vi "GetMatchNum.vi"(7 "Update?":bool, 8 "MatchNumberIn":u16) -> (3 "MatchNumberOut":u16)   [LabVIEW 2017]
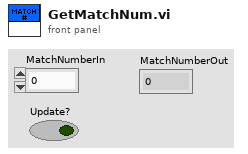
[diagram p1: front panel]
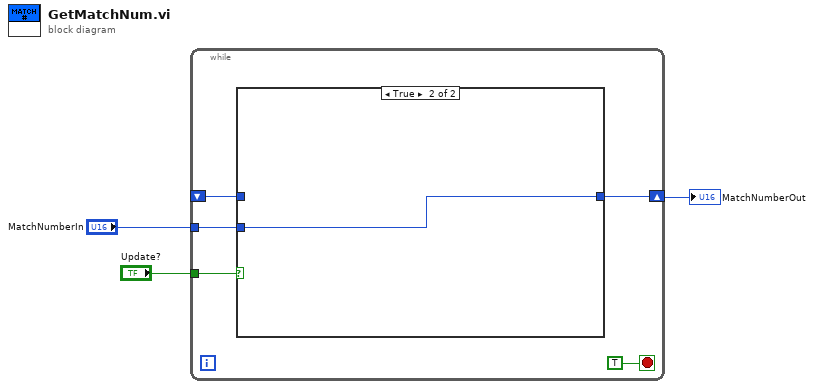
[diagram p0: block diagram]
diagram:
  n1 = while {
    shift-right: [w7] -> w1
    shift-left: _ -> [w8]
    tunnel: "MatchNumberIn" -> [w6]
    tunnel: "Update?" -> [w5]
    stop <- TRUE stop-if-true
    n2 = case shown="True" w5 {
      tunnel: w8 -> [w9 _]
      tunnel: [w9 w10] -> w7
      tunnel: w6 -> [_ w10]
      frame False {
      }
      frame True {
      }
    }
  }
  "MatchNumberOut" <- w1
